vi "Browse_Disk_Sever.vi"(1 "Folder Hierarchy":string[](array[string])) -> (0 "Folders and files":T1(array[cluster]))   [LabVIEW 2012]
uses:
  Anemometry/Anemometry Sub Vis/Globals/Constants_global.vi
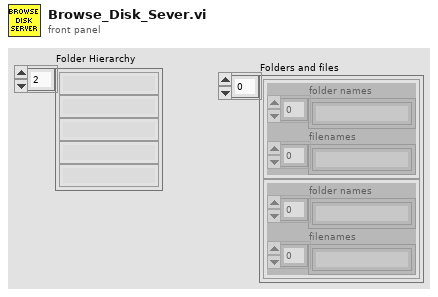
[diagram p1: front panel]
types:
  T1 = cluster{"folder names":string[], "filenames":string[]}[]
  T2 = cluster{"folder names":string[], "filenames":string[]}
  T3 = cluster{"Files Out":string[], "Files Out":string[]}
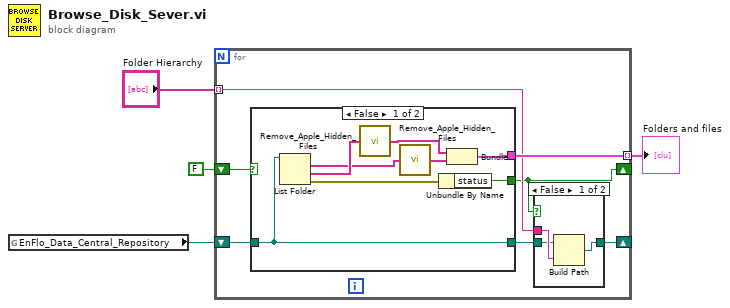
[diagram p0: block diagram]
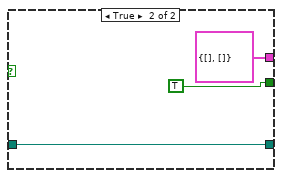
[diagram p3: hidden frame]
diagram:
  n1 = global read "Constants_global.vi" "EnFlo_Data_Central_Repository"() -> (w1:path)
  n2 = for {
    shift-right: [w6] -> _
    shift-left: w1 -> [w9]
    tunnel: [w11] -> w4 mode=indexing
    shift-right: [w5] -> _
    shift-left: FALSE -> [w10]
    tunnel: "Folder Hierarchy" -> [w8] mode=indexing
    n3 = case shown="False" w10 {
      tunnel: w9 -> [w20 w24]
      tunnel: [w20 w24] -> w7
      tunnel: [w23 T2 {"folder names"=[], "filenames"=[]}] -> w11
      tunnel: [w21 TRUE ("status")] -> w5
      frame False {
        n4 = List Folder(path=w20) -> (filenames=w17:string[], folder names=w19:string[], error out=w22:errorcluster)  [unwired: 3 in, 1 out]
        n5 = call "Remove_Apple_Hidden_Files.vi"("Files In"=w19) -> ("Files Out"=w18:string[])
        n6 = call "Remove_Apple_Hidden_Files.vi"("Files In"=w17) -> ("Files Out"=w16:string[])
        n7 = Unbundle By Name(w22) -> ("status"=w21:bool)
        n8 = Bundle("Files Out"=w18, "Files Out"=w16) -> (w23:T3)  [unwired: 1 in]
      }
      frame True {
      }
    }
    n9 = case shown="False" w5 {
      tunnel: w8 -> [w14 _]
      tunnel: w7 -> [w13 w15]
      tunnel: [w12 w15] -> w6
      frame False {
        n10 = Build Path(base path=w13, name or relative path=w14) -> (appended path=w12:path)
      }
      frame True {
      }
    }
  }
  "Folders and files" <- w4
